vi "muCTA_EnFlo_Specific.vi"(6 "N samples":u32, 7 "VISA resource name":refnum<visa-resource-name>) -> (0 "I/O error":errorcluster, 1 "% chk err.":dbl, 3 "Data out":sgl[][](array[numeric]))   [LabVIEW 2018]
uses:
  ctls/muCTA_USB Tx msg cluster.ctl
panel:
  out "N samples acq.":u32
  out "loop dt (s)":dbl format="%#_2g"
  out "Time history":cluster{sgl, "Sample interval (s)":sgl, sgl[][]}(graph)
  in  "Stop":bool
  # "Sampling rate fixed at 100 Hz\n(for now)"
  # "\"Data out\" array ordered as below"
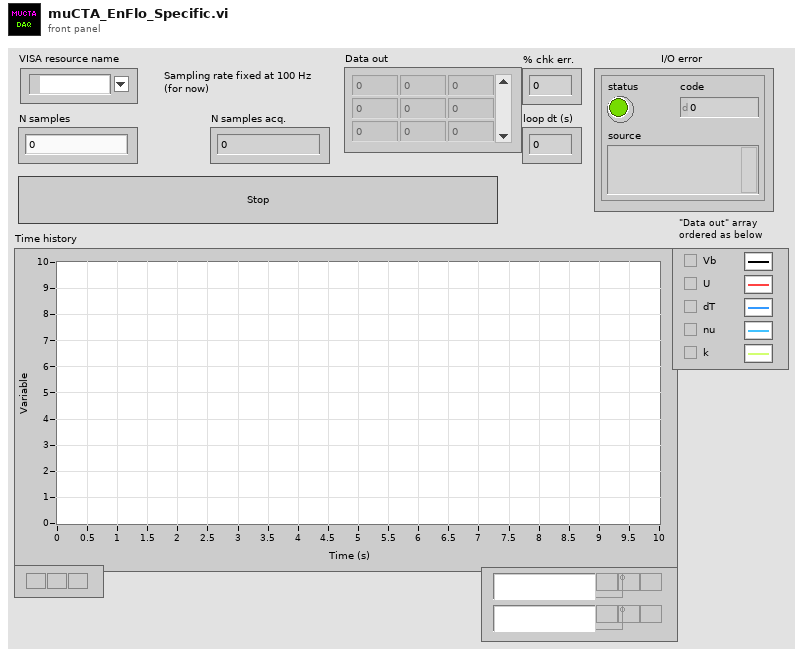
[diagram p1: front panel]
types:
  T1 = typedef "muCTA_USB Tx msg cluster.ctl" = cluster{"dest":u8, "A/D/C/I":string, "R/W":string, "chan":u8, "val (float)":sgl}
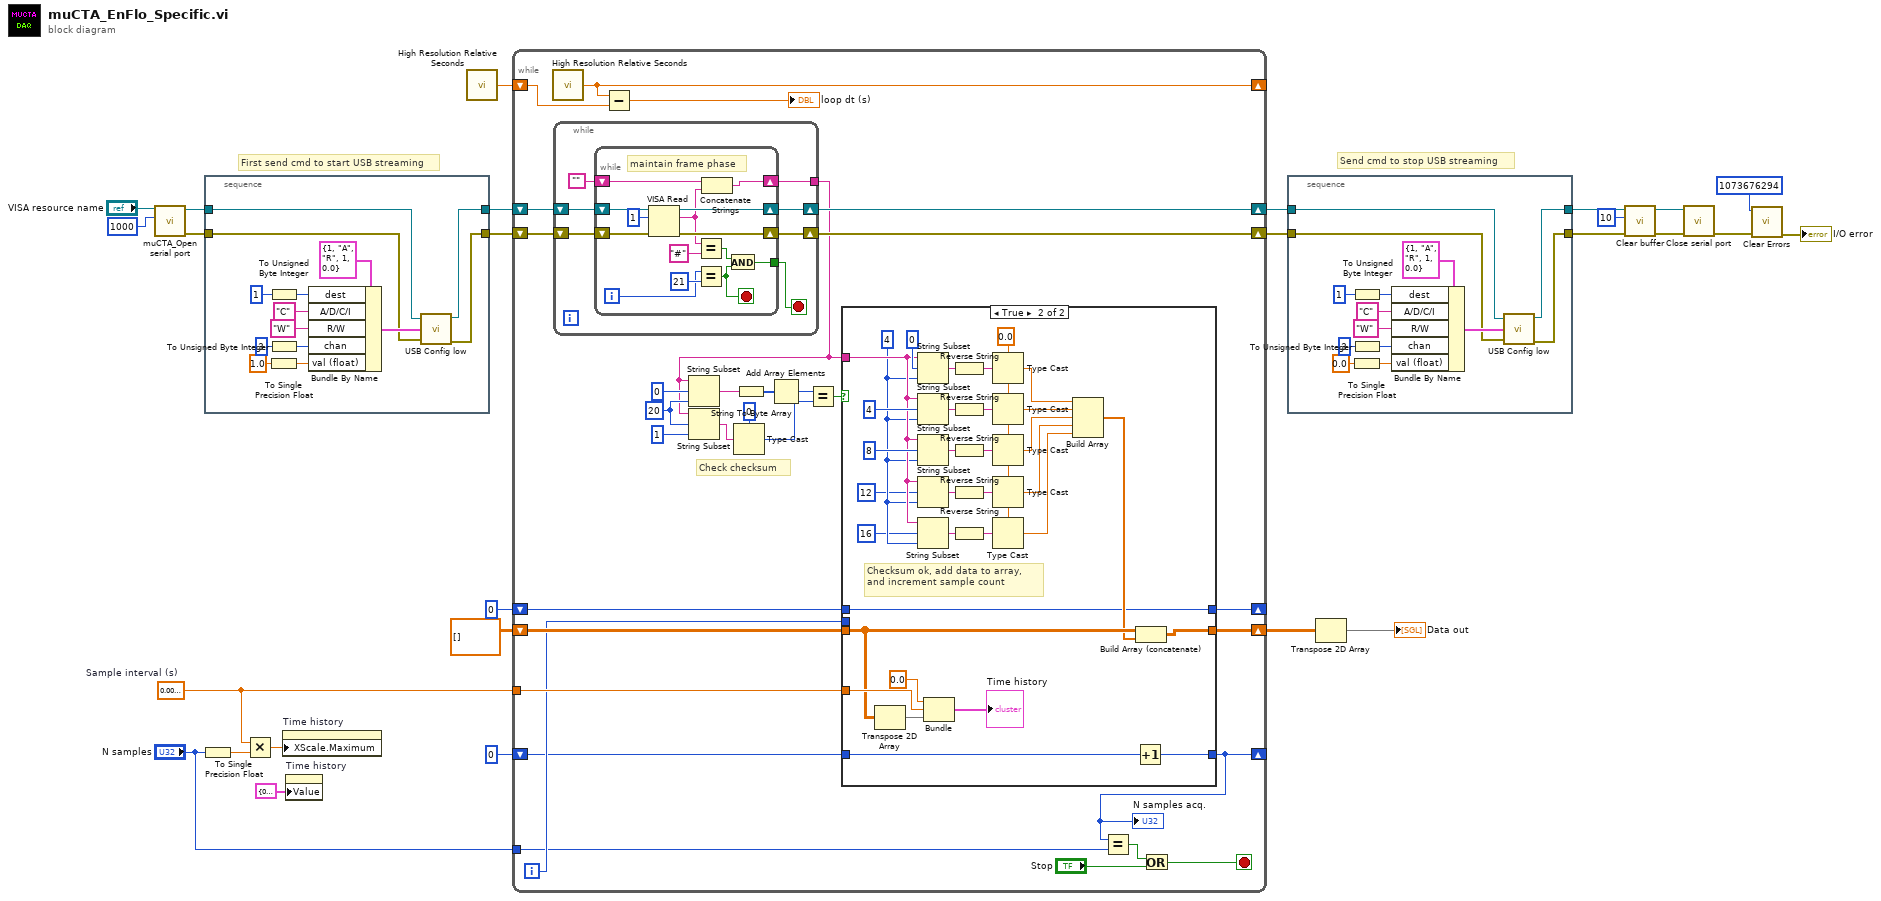
[diagram p0: block diagram]
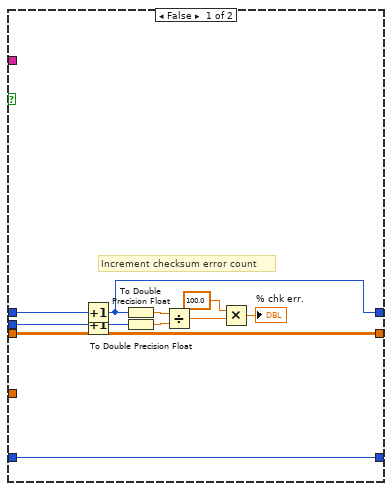
[diagram p2: hidden frame]
diagram:
  w6 = sgl 0.01  # Sample interval (s)
  # "Send cmd to stop USB streaming"
  # "First send cmd to start USB streaming"
  n1 = call "muCTA_Open serial port.vi"("timeout (ms)"=u32 1000, "VISA resource name"="VISA resource name") -> ("Error out"=w22:errorcluster, "VISA resource name out"=w18:refnum<visa-resource-name>)  [unwired: 8 in]
  n2 = To Single Precision Float(number="N samples") -> (single precision float=w7:sgl)
  n3 = stacked-sequence {
    tunnel: w18 -> [w30]
    tunnel: [w31] -> w21
    tunnel: w22 -> [w29]
    tunnel: [w28] -> w17
    frame #0 {
      n4 = To Unsigned Byte Integer(number=u8 1 ("Address")) -> (unsigned 8bit integer=w36:u8)
      n5 = To Unsigned Byte Integer(number=u8 3) -> (unsigned 8bit integer=w35:u8)
      n6 = To Single Precision Float(number=sgl 1.0) -> (single precision float=w38:sgl)
      n7 = Bundle By Name(cluster=T1 {"dest"=1, "A/D/C/I"="A", "R/W"="R", "chan"=1, "val (float)"=0.0} ("Tx msg cluster"), "dest"=w36, "A/D/C/I"="C" ("A/D"), "R/W"="W", "chan"=w35, "val (float)"=w38) -> (w37:T1)
      n8 = call "USB Config low.vi"("Port"=w30, "Tx msg cluster"=w37, "Error in"=w29) -> ("Port out"=w28:refnum<visa-resource-name>, "Error out"=w31:errorcluster)  [unwired: 1 in, 1 out]
    }
  }
  n9 = Multiply(x=w6, y=w7) -> (x*y=w5:sgl)
  n10 = property on="Time history" class="WFGraph (strict)"("XScale.Maximum"=w5) -> ()  [unwired: 2 in, 2 out]
  n11 = property on="Time history" class="WFGraph (strict)"("Value"=cluster{sgl, "Sample interval (s)":sgl, sgl[][]} {0.0, "Sample interval (s)"=0.0, []} ("Time history")) -> ()  [unwired: 2 in, 2 out]
  n12 = call <vilib>:"High Resolution Relative Seconds.vi"() -> ("relative seconds"=w25:dbl)
  n13 = while {
    shift-right: [w69] -> w19
    shift-left: w21 -> [w70]
    shift-right: [w68] -> w20
    shift-left: w17 -> [w71]
    shift-right: [w49] -> w2
    shift-left: sgl[][] [] -> [w65]
    tunnel: w6 -> [w66]
    shift-right: [w53] -> _
    shift-left: u32 0 -> [w54]
    shift-right: [w51] -> _
    shift-left: w25 -> [w50]
    tunnel: "N samples" -> [w43]
    shift-right: [w44] -> _
    shift-left: u32 0 -> [w45]
    i -> [w46]
    stop <- w47 stop-if-true
    w58 = 20 ("length (rest)")
    # "Check checksum"
    n14 = call <vilib>:"High Resolution Relative Seconds.vi"() -> ("relative seconds"=w51:dbl)
    n15 = while {
      shift-right: [w75] -> w68
      shift-left: w71 -> [w78]
      shift-right: [w76] -> w69
      shift-left: w70 -> [w77]
      tunnel: [w72] -> w55
      stop <- w73 stop-if-true
      n16 = while {
        shift-right: [w88] -> w75
        shift-left: w78 -> [w92]
        shift-right: [w89] -> w76
        shift-left: w77 -> [w91]
        shift-right: [w83] -> w72
        shift-left: "" -> [w82]
        tunnel: [w79] -> w73
        i -> [w85]
        stop <- w80 stop-if-true
        # "maintain frame phase"
        n17 = VISA Read(VISA resource name=w92, byte count=u32 1, error in (no error)=w91) -> (VISA resource name out=w88:refnum<visa-resource-name>, read buffer=w81:string, error out=w89:errorcluster)  [unwired: 1 out]
        n18 = Equal?(x=w81, y="#" ("search string/char (-)")) -> (x = y?=w84:bool)
        n19 = Equal?(x=w85, y=21) -> (x = y?=w80:bool)
        n20 = Concatenate Strings(w82, w81) -> (w83:string)
        n21 = And(x=w84, y=w80) -> (x .and. y?=w79:bool)
      }
    }
    n22 = Subtract(x=w51, y=w50) -> (x-y=→"loop dt (s)":dbl)
    n23 = String Subset(string=w55, offset (0)=0, length (rest)=w58) -> (substring=w62:string)
    n24 = String Subset(string=w55, offset (0)=w58, length (rest)=1 ("length (rest)")) -> (substring=w60:string)
    n25 = Type Cast(type=u8 0, x=w60) -> (*(type *) &x=w56:u8)
    n26 = String To Byte Array(string=w62) -> (unsigned byte array=w61:u8[])
    n27 = Add Array Elements(numeric array=w61) -> (sum=w57:u8)
    n28 = Equal?(x=w57, y=w56) -> (x = y?=w67:bool)
    n29 = case shown="True" w67 {
      tunnel: w55 -> [_ w112]
      tunnel: [w103 w128] -> w49
      tunnel: w65 -> [w103 w125]
      tunnel: w66 -> [_ w126]
      tunnel: w54 -> [w102 w120]
      tunnel: w46 -> [w101 _]
      tunnel: [w96 w120] -> w53
      tunnel: [w93 w105] -> w44
      tunnel: w45 -> [w93 w104]
      frame False {
        # "Increment checksum error count"
        n30 = Increment(x=w102) -> (x+1=w96:u32)
        n31 = Increment(x=w101) -> (x+1=w94:i32)
        n32 = To Double Precision Float(number=w96) -> (double precision float=w99:dbl)
        n33 = To Double Precision Float(number=w94) -> (double precision float=w100:dbl)
        n34 = Divide(x=w99, y=w100) -> (x/y=w98:dbl)
        n35 = Multiply(x=100.0, y=w98) -> (x*y=→"% chk err.":dbl)
      }
      frame True {
        w111 = sgl 0.0
        w108 = 4 ("length (rest)")
        # "Checksum ok, add data to array, and increment sample count"
        n36 = Transpose 2D Array(2D array=w125) -> (transposed array=w124:sgl[][])
        n37 = String Subset(string=w112, offset (0)=0, length (rest)=w108) -> (substring=w136:string)
        n38 = String Subset(string=w112, offset (0)=4 ("length (rest)"), length (rest)=w108) -> (substring=w133:string)
        n39 = String Subset(string=w112, offset (0)=8 ("length (rest)"), length (rest)=w108) -> (substring=w113:string)
        n40 = String Subset(string=w112, offset (0)=12 ("length (rest)"), length (rest)=w108) -> (substring=w114:string)
        n41 = String Subset(string=w112, offset (0)=16 ("length (rest)"), length (rest)=w108) -> (substring=w117:string)
        n42 = Bundle(sgl 0.0, "Sample interval (s)"=w126, w124) -> (→"Time history":cluster{sgl, "Sample interval (s)":sgl, sgl[][]})  [unwired: 1 in]
        n43 = Reverse String(1:w136) -> (0:w135:string)
        n44 = Reverse String(1:w133) -> (0:w134:string)
        n45 = Reverse String(1:w113) -> (0:w122:string)
        n46 = Reverse String(1:w114) -> (0:w115:string)
        n47 = Reverse String(1:w117) -> (0:w116:string)
        n48 = Type Cast(type=w111, x=w135) -> (*(type *) &x=w131:sgl)
        n49 = Type Cast(type=w111, x=w134) -> (*(type *) &x=w130:sgl)
        n50 = Type Cast(type=w111, x=w122) -> (*(type *) &x=w121:sgl)
        n51 = Type Cast(type=w111, x=w115) -> (*(type *) &x=w110:sgl)
        n52 = Type Cast(type=w111, x=w116) -> (*(type *) &x=w109:sgl)
        n53 = Build Array(w131, w130, w121, w110, w109) -> (w123:sgl[])
        n54 = Increment(x=w104) -> (x+1=w105:u32)
        n55 = Build Array (concatenate)(w125, w123) -> (w128:sgl[][])
      }
    }
    "N samples acq." <- w44
    n56 = Equal?(x=w44, y=w43) -> (x = y?=w42:bool)
    n57 = Or(x=w42, y="Stop") -> (x .or. y?=w47:bool)
  }
  n58 = stacked-sequence {
    tunnel: w20 -> [w138]
    tunnel: [w140] -> w15
    tunnel: [w137] -> w16
    tunnel: w19 -> [w139]
    frame #0 {
      n59 = To Unsigned Byte Integer(number=u8 1 ("Address")) -> (unsigned 8bit integer=w145:u8)
      n60 = To Unsigned Byte Integer(number=u8 3) -> (unsigned 8bit integer=w144:u8)
      n61 = To Single Precision Float(number=sgl 0.0) -> (single precision float=w147:sgl)
      n62 = Bundle By Name(cluster=T1 {"dest"=1, "A/D/C/I"="A", "R/W"="R", "chan"=1, "val (float)"=0.0} ("Tx msg cluster"), "dest"=w145, "A/D/C/I"="C" ("A/D"), "R/W"="W", "chan"=w144, "val (float)"=w147) -> (w146:T1)
      n63 = call "USB Config low.vi"("Port"=w138, "Tx msg cluster"=w146, "Error in"=w139) -> ("Port out"=w137:refnum<visa-resource-name>, "Error out"=w140:errorcluster)  [unwired: 1 in, 1 out]
    }
  }
  n64 = Transpose 2D Array(2D array=w2) -> (transposed array=→"Data out":sgl[][])
  n65 = call "Clear buffer.vi"("Error in"=w15, "dt for timeout (ms)"=u32 10, "VISA resource name in"=w16) -> ("Error out"=w14:errorcluster, "VISA resource name out"=w13:refnum<visa-resource-name>)  [unwired: 3 in]
  n66 = call "Close serial port.vi"("Error in"=w14, "VISA resource name"=w13) -> ("Error out"=w10:errorcluster)  [unwired: 9 in]
  n67 = call <vilib>:"Clear Errors.vi"("error in (no error)"=w10, "specific error code to clear (0: all)"=1073676294) -> ("error out"=→"I/O error":errorcluster)  [unwired: 4 in, 1 out]
